vi "Update Cell.vi"(9 "Col":i32, 10 "Row":i32, 11 "Heat Map in":refnum<class "Heat Map.lvclass">) -> (3 "Heat Map out":refnum<class "Heat Map.lvclass">)   [LabVIEW 2021, in "Heat Map.lvclass"]
uses:
  Heat Map.lvclass
  Heat Map.lvclass/Heat Map.ctl
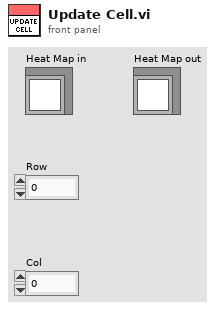
[diagram p1: front panel]
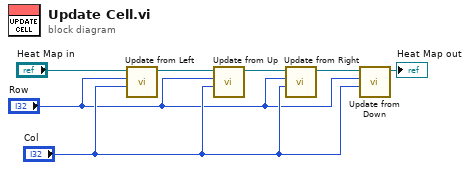
[diagram p0: block diagram]
diagram:
  n1 = call "Update from Left.vi"("Col"="Col", "Row"="Row", "Proto in"="Heat Map in") -> ("Proto out"=w2:refnum<class "Heat Map.lvclass">)  [unwired: 8 in]
  n2 = call "Update from Up.vi"("Col"="Col", "Row"="Row", "Proto in"=w2) -> ("Proto out"=w3:refnum<class "Heat Map.lvclass">)  [unwired: 8 in]
  n3 = call "Update from Right.vi"("Col"="Col", "Row"="Row", "Proto in"=w3) -> ("Proto out"=w4:refnum<class "Heat Map.lvclass">)  [unwired: 8 in]
  n4 = call "Update from Down.vi"("Col"="Col", "Row"="Row", "Proto in"=w4) -> ("Proto out"=→"Heat Map out":refnum<class "Heat Map.lvclass">)  [unwired: 8 in]
